vi "Inline Vims in VI.vi"(4 "Just Fixup":bool, 8 "error in (no error)":errorcluster, 10 "References":refnum<vi>[](array[refnum]), 11 "VI in":refnum<vi>) -> (0 "error out":errorcluster, 1 "Nothing to Inline":bool, 3 "VI out":refnum<vi>)   [LabVIEW 2020, in "vim-liner.lvlib"]
uses:
  vim-liner.lvlib
  bbb8ce3b-7b85-409e-92b0-40d252696f7c.vi
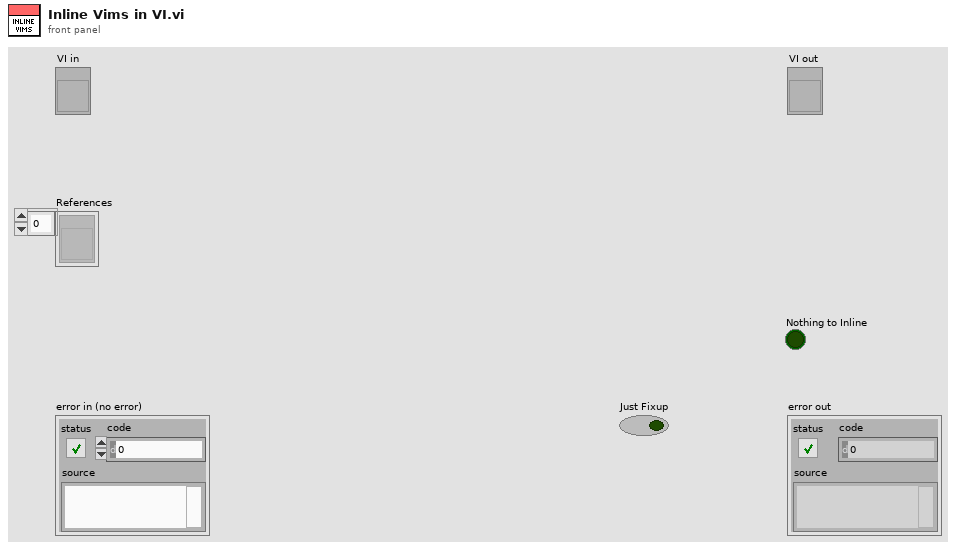
[diagram p1: front panel]
types:
  T1 = enum32{"Invalid", "Standard", "Closed", "Hidden", "Minimized", "Maximized"}
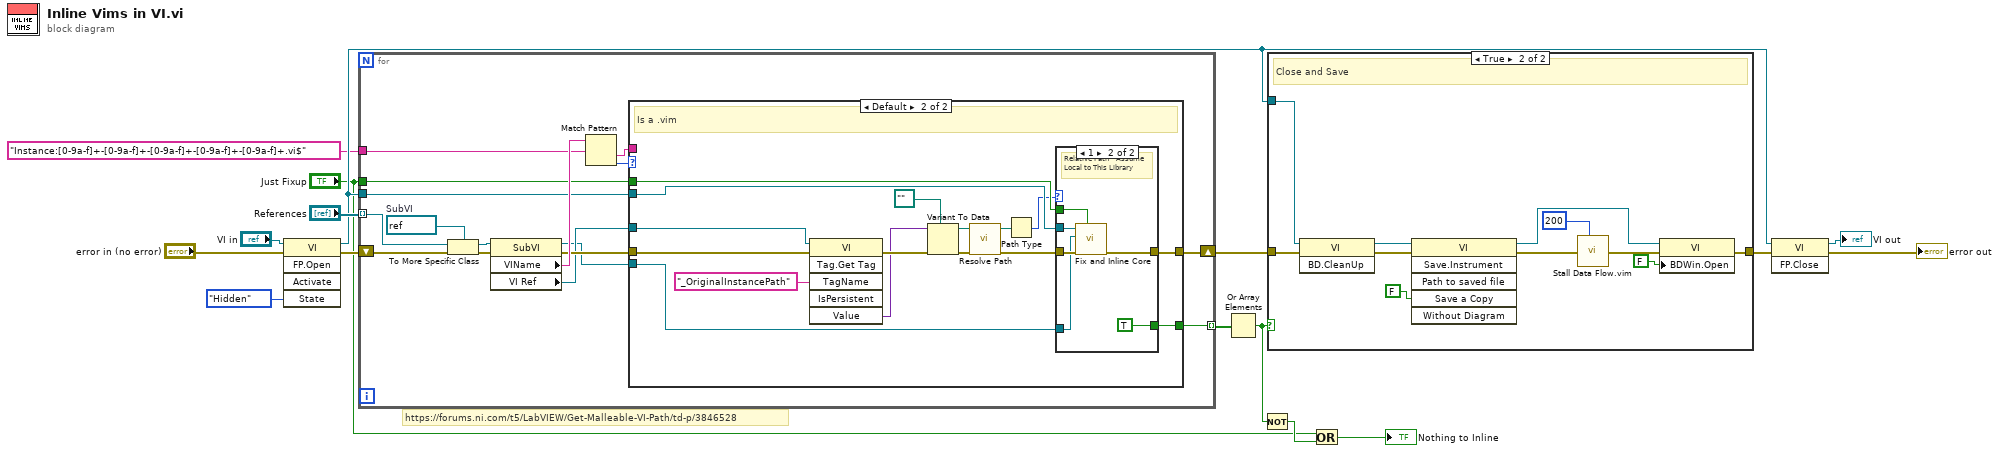
[diagram p0: block diagram]
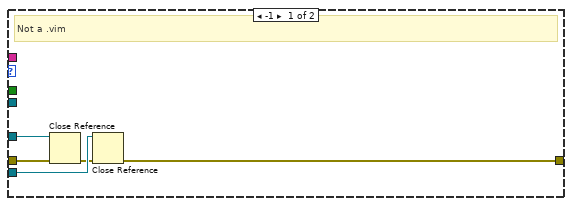
[diagram p3: hidden frame]
diagram:
  # "https://forums.ni.com/t5/LabVIEW/Get-Malleable-VI-Path/td-p/3846528"
  n1 = invoke class="VI" method="FP.Open"(reference="VI in", error in="error in (no error)", "State"=T1."Hidden") -> (reference out=w8:refnum<vi>, error out=w15:errorcluster)  [unwired: 2 in, 3 out]
  n2 = for {
    shift-right: [w25] -> w11
    shift-left: w15 -> [w32]
    tunnel: "References" -> [w31] mode=indexing
    tunnel: w8 -> [w24]
    tunnel: [w23] -> w12 mode=indexing
    tunnel: "Instance:[0-9a-f]+-[0-9a-f]+-[0-9a-f]+-[0-9a-f]+-[0-9a-f]+.vi$" ("regular expression") -> [w20]
    tunnel: "Just Fixup" -> [w17]
    w30 = refnum<vi> refnum  # SubVI
    n3 = To More Specific Class(target class=w30, reference=w31, error in=w32) -> (specific class reference=w29:refnum<vi>, error out=w28:errorcluster)
    n4 = property class="SubVI"(reference=w29, error in=w28) -> (reference out=w18:refnum<vi>, error out=w22:errorcluster, "VIName"=w26:string, "VI Ref"=w19:refnum<vi>)
    n5 = Match Pattern(string=w26, regular expression=w20) -> (after substring=w27:string, offset past match=w21:i32)  [unwired: 1 in, 2 out]
    n6 = case shown="Default" w21 {
      tunnel: w27 -> [_ _]
      tunnel: [w37 w53] -> w25
      tunnel: w19 -> [w35 w45]
      tunnel: w24 -> [_ w52]
      tunnel: [_ w51] -> w23
      tunnel: w22 -> [w33 w46]
      tunnel: w18 -> [w36 w50]
      tunnel: w17 -> [_ w42]
      frame -1 {
        # "Not a .vim"
        n7 = Close Reference(reference=w35, error in (no error)=w33) -> (error out=w34:errorcluster)
        n8 = Close Reference(reference=w36, error in (no error)=w34) -> (error out=w37:errorcluster)
      }
      frame Default {
        # "Is a .vim"
        n9 = invoke class="VI" method="Tag.Get Tag"(reference=w45, error in=w46, "TagName"="_OriginalInstancePath" ("Tag Name")) -> (error out=w49:errorcluster, "Value"=w48:variant)  [unwired: 3 in, 4 out]
        n10 = Variant To Data(error in=w49, type=path "", Variant=w48) -> (data=w40:path, error out=w44:errorcluster)
        n11 = call "Resolve Path.vi"("error in (no error)"=w44, "Path"=w40) -> ("error out"=w41:errorcluster, "Resolved"=w39:path)  [unwired: 8 in]
        n12 = Path Type(1:w39) -> (0:w38:i16)
        n13 = case shown="1" w38 {
          tunnel: w52 -> [_ w60]
          tunnel: [w54 w59] -> w53
          tunnel: [_ TRUE] -> w51
          tunnel: w41 -> [w54 w57]
          tunnel: w50 -> [_ w56]
          tunnel: w42 -> [_ w55]
          frame Default {
          }
          frame 1 {
            # "Relative Path - Assume Local to This Library"
            n14 = call "Fix and Inline Core.vi"("Just Fixup"=w55, "error in (no error)"=w57, "SubVI Refnum in"=w56, "VI in"=w60) -> ("error out"=w59:errorcluster)  [unwired: 7 in]
          }
        }
      }
    }
  }
  n15 = Or Array Elements(Boolean array=w12) -> (logical OR=w10:bool)
  n16 = Not(x=w10) -> (.not. x?=w3:bool)
  n17 = case shown="True" w10 {
    tunnel: w8 -> [_ w72]
    tunnel: w11 -> [w61 w71]
    tunnel: [w61 w65] -> w9
    frame False {
      # "No Updates"
    }
    frame True {
      # "Close and Save"
      n18 = invoke class="VI" method="BD.CleanUp"(reference=w72, error in=w71) -> (reference out=w69:refnum<vi>, error out=w68:errorcluster)  [unwired: 1 in, 1 out]
      n19 = invoke class="VI" method="Save.Instrument"(reference=w69, error in=w68, "Save a Copy"=FALSE) -> (reference out=w66:refnum<vi>, error out=w67:errorcluster)  [unwired: 3 in, 4 out]
      n20 = call "Stall Data Flow.vim"("value in"=w67, "milliseconds to wait"=u32 200) -> ("value out"=w63:errorcluster)  [unwired: 1 out]
      n21 = property class="VI"(reference=w66, error in=w63, "BDWin.Open"=FALSE ("Block Diagram Window:Open")) -> (error out=w65:errorcluster)  [unwired: 1 out]
    }
  }
  n22 = Or(x="Just Fixup", y=w3) -> (x .or. y?=→"Nothing to Inline":bool)
  n23 = invoke class="VI" method="FP.Close"(reference=w8, error in=w9) -> (reference out=→"VI out":refnum<vi>, error out=→"error out":errorcluster)  [unwired: 1 in, 1 out]
